vi "Get All Scanner Rotations.vi"(11 "Scanner":T2) -> (3 "Scanner Rotations":T1(array[cluster]))   [LabVIEW 2021]
uses:
  <vilib>/Analysis/coordinate.llb/3D Cartesian Coordinate Rotation (Direction) (Array).vi
  <vilib>/Analysis/NI_AALPro.lvlib
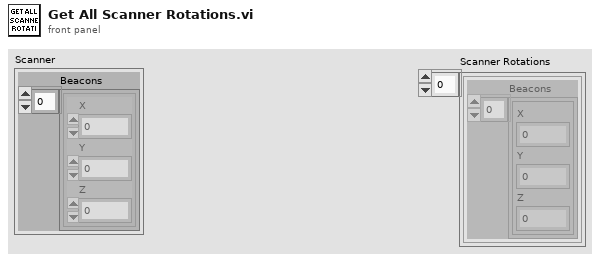
[diagram p1: front panel]
types:
  T1 = cluster{"Beacons":cluster{"X":i64, "Y":i64, "Z":i64}[]}[]
  T2 = cluster{"Beacons":cluster{"X":i64, "Y":i64, "Z":i64}[]}
  T3 = typedef "NI_Matrix.lvlib/RealMatrix.ctl" = dbl[][]
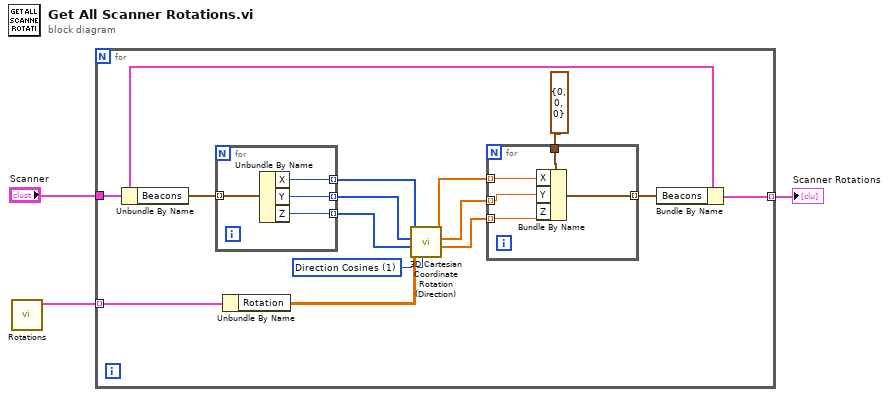
[diagram p0: block diagram]
diagram:
  n1 = call "Rotations.vi"() -> ("Rotations"=w1:cluster{"Rotation":T3}[])  [unwired: 11 in]
  n2 = for {
    tunnel: "Scanner" -> [w9]
    tunnel: [w7] -> w2 mode=indexing
    tunnel: w1 -> [w6] mode=indexing
    w4 = u16 1 items=["Direction Angles", "Direction Cosines"] ("rotation matrix type")
    n3 = Unbundle By Name(w9) -> ("Beacons"=w17:cluster{"X":i64, "Y":i64, "Z":i64}[])
    n4 = for {
      tunnel: w17 -> [w26] mode=indexing
      tunnel: [w25] -> w16 mode=indexing
      tunnel: [w24] -> w15 mode=indexing
      tunnel: [w23] -> w14 mode=indexing
      n5 = Unbundle By Name(w26) -> ("X"=w25:i64, "Y"=w24:i64, "Z"=w23:i64)
    }
    n6 = Unbundle By Name(w6) -> ("Rotation"=w5:T3)
    n7 = call-poly <vilib>:"3D Cartesian Coordinate Rotation (Direction).vi"("rotation matrix type"=w4, "Rotation Matrix"=w5, "Z"=w14, "Y"=w15, "X"=w16) -> ("Z Out"=w11:dbl[], "Y Out"=w12:dbl[], "X Out"=w13:dbl[])  [unwired: 3 in, 1 out]
    n8 = for {
      tunnel: w13 -> [w19] mode=indexing
      tunnel: w12 -> [w20] mode=indexing
      tunnel: w11 -> [w21] mode=indexing
      tunnel: cluster{"X":i64, "Y":i64, "Z":i64} {"X"=0, "Y"=0, "Z"=0} -> [w22]
      tunnel: [w18] -> w8 mode=indexing
      n9 = Bundle By Name(cluster=w22, "X"=w19, "Y"=w20, "Z"=w21) -> (w18:cluster{"X":i64, "Y":i64, "Z":i64})
    }
    n10 = Bundle By Name(cluster=w9, "Beacons"=w8) -> (w7:T2)
  }
  "Scanner Rotations" <- w2
